vi "get Temperature LV.vi"(8 "error in (no error)":errorcluster, 10 "status":u32, 11 "temperature":i32) -> (0 "error out":errorcluster, 2 "status out":u32, 3 "temperature out":i32)   [LabVIEW 2016, in "cameraLibrary.lvlib"]
doc: "Returns the current camera array temperature.\n\n\nvoid CAMERALIBRARYSHARED_EXPORT getTemperatureLV(int *temperature, unsigned int *status);"
uses:
  cameraLibrary.lvlib
  cameraLibrary.dll
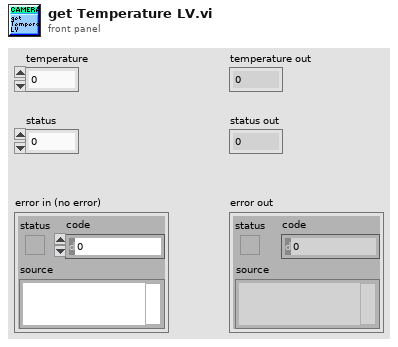
[diagram p1: front panel]
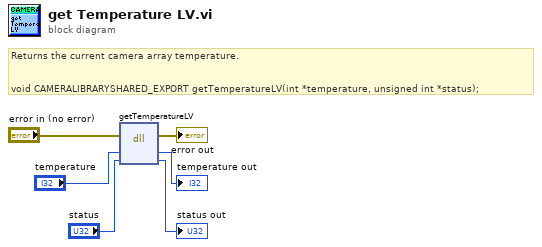
[diagram p0: block diagram]
diagram:
  # "Returns the current camera array temperature.\n\n\nvoid CAMERALIBRARYSHARED_EXPORT getTemperatureLV(int *temperature, unsigned int *status);"
  n1 = dll-call lib="C:/Users/TMM/repos/EXPRES/FEM/FTT/support/Camera Library/cameraLibrary.*" fn="getTemperatureLV"(error in="error in (no error)", "temperature"="temperature", "status"="status") -> (error out=→"error out":errorcluster, "temperature"=→"temperature out":i32, "status"=→"status out":u32)  [unwired: 3 in, 1 out]
